vi "Space Constant.vi"() -> (0 "String":string)   [LabVIEW 2017]
doc: "Use this constant to supply a one-character space string to the block diagram."
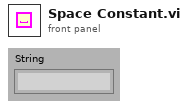
[diagram p1: front panel]
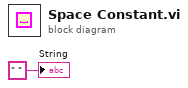
[diagram p0: block diagram]
diagram:
  "String" <- " "
